vi "startShooting.vi"(8 "error in (no error)":errorcluster, 11 "ICCameraController in":refnum<class "ICCameraController.lvclass">) -> (0 "error out":errorcluster, 1 "Warning Message":string, 2 "Final Acquisition Timings":T1, 3 "ICCameraController out":refnum<class "ICCameraController.lvclass">)   [LabVIEW 2011, in "Hardware.lvlib" / "Channels.lvlib" / "ICCameraController.lvclass"]
uses:
  ICCameraController.lvclass
  ICCameraAcquisitor/ICCameraAcquisitor.lvclass
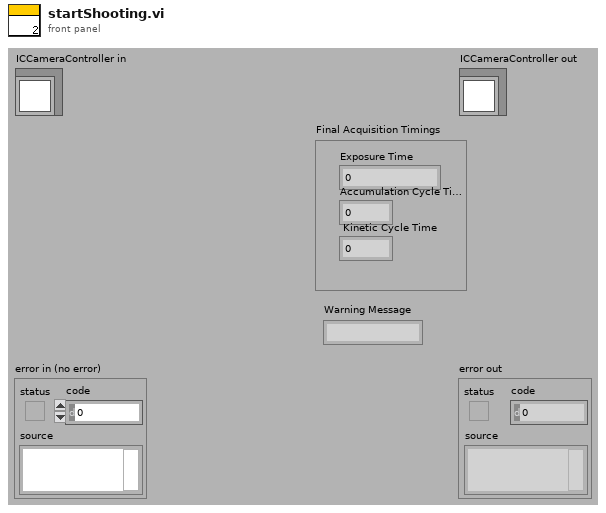
[diagram p1: front panel]
types:
  T1 = cluster{"Exposure Time":dbl, "Accumulation Cycle Time":dbl, " Kinetic Cycle Time":dbl}
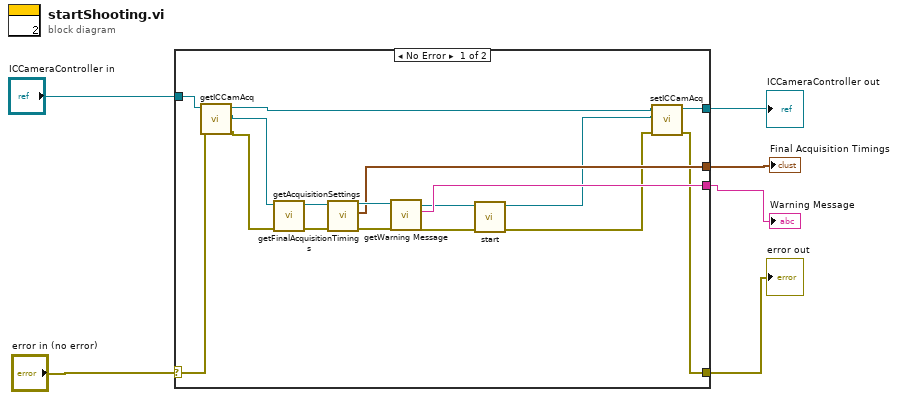
[diagram p0: block diagram]
diagram:
  n1 = case shown="No Error" "error in (no error)" {
    selector: "error in (no error)" -> [w14 w25]
    tunnel: [w7 w25] -> w4
    tunnel: [w10 w24] -> w5
    tunnel: [w19 _] -> w3
    tunnel: [w18 _] -> w2
    tunnel: "ICCameraController in" -> [w15 w24]
    frame No Error {
      n2 = call-dynamic "getICCamAcq.vi"("error in (no error)"=w14, "ICCameraController in"=w15) -> ("error out"=w12:errorcluster, "ICCameraAcquisitor"=w13:refnum<class "ICCameraAcquisitor.lvclass">, "ICCameraController out"=w11:refnum<class "ICCameraController.lvclass">)  [unwired: 7 in]
      n3 = call-dynamic "getAcquisitionSettings.vi"("error in (no error)"=w12, "CameraAcquisitor in"=w13) -> ("error out"=w22:errorcluster, "CameraAcquisitor out"=w23:refnum<class "ICCameraAcquisitor.lvclass">)  [unwired: 8 in]
      n4 = call-dynamic "getFinalAcquisitionTimings.vi"("error in (no error)"=w22, "ICCameraAcquisitor.lvclass in"=w23) -> ("error out"=w20:errorcluster, "Final Acquisition Timings"=w19:T1, "ICCameraAcquisitor.lvclass out"=w21:refnum<class "ICCameraAcquisitor.lvclass">)  [unwired: 7 in]
      n5 = call-dynamic "getWarning Message.vi"("error in (no error)"=w20, "CameraAcquisitor.lvclass in"=w21) -> ("error out"=w17:errorcluster, "Warning Message"=w18:string, "CameraAcquisitor.lvclass out"=w16:refnum<class "ICCameraAcquisitor.lvclass">)  [unwired: 7 in]
      n6 = call-dynamic "start.vi"("error in (no error)"=w17, "ICCameraAcquisitor in"=w16) -> ("error out"=w8:errorcluster, "ICCameraAcquisitor out"=w9:refnum<class "ICCameraAcquisitor.lvclass">)  [unwired: 8 in]
      n7 = call-dynamic "setICCamAcq.vi"("error in (no error)"=w8, "ICCameraAcquisitor"=w9, "ICCameraController in"=w11) -> ("error out"=w7:errorcluster, "ICCameraController out"=w10:refnum<class "ICCameraController.lvclass">)  [unwired: 7 in]
    }
    frame Error {
    }
  }
  "error out" <- w4
  "ICCameraController out" <- w5
  "Final Acquisition Timings" <- w3
  "Warning Message" <- w2
